vi "Add Library to Project.vi"   [LabVIEW 2011, in "Generator.lvlib"]
uses:
  Generator.lvlib
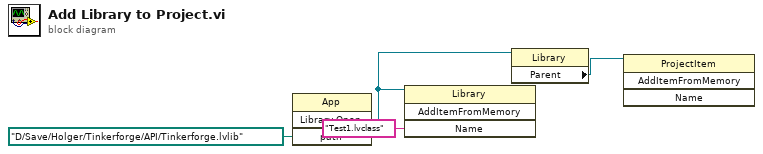
[diagram p0: block diagram]
diagram:
  n1 = invoke class="App" method="Library.Open"("path"=path "D:/Save/Holger/Tinkerforge/API/Tinkerforge.lvlib" ("Path")) -> ("Open Library"=w2:refnum<vi>)  [unwired: 3 in, 3 out]
  n2 = invoke class="Library" method="AddItemFromMemory"(reference=w2, "Name"="Test1.lvclass") -> ()  [unwired: 2 in, 4 out]
  n3 = property class="Library"(reference=w2) -> ("Parent"=w1:refnum<vi>)  [unwired: 1 in, 2 out]
  n4 = invoke class="ProjectItem" method="AddItemFromMemory"(reference=w1) -> ()  [unwired: 3 in, 4 out]
